vi "Configure Scaling.vi"(0 "Plugin_UI in":refnum<class "Plugin_UI.lvclass">, 11 "error in (no error)":errorcluster, 12 "Selected Channel":string) -> (4 "Plugin_UI out":refnum<class "Plugin_UI.lvclass">, 6 "Scale Active?":bool, 15 "error out":errorcluster)   [LabVIEW 2020, in "Plugin.lvlib" / "Plugin_UI.lvclass"]
doc: "Extracts all the measurement channels and display it in the Scale Settings window. Once the Scale settings window is closed, the scalling information of all the active channel is replaced with latest information from Scale Settings VI."
uses:
  Plugin_UI.lvclass
  C:/SVN_LabSys/labsys_lvcode/LabSys_SourceCode/builds/Libraries/LabSys Framework.lvlibp/Configurable Data Node/Configuration Interface/Configuration Interface.lvclass
  Plugin_UI.lvclass/Plugin_UI.ctl
  Read Input Channels[].vi
  Write Input Channels[].vi
  builds/Libraries/LabSys Framework.lvlibp/Configurable Data Node/Configuration Interface/Read Module Configuration.vi
  Read Scaling Functions.vi
  Read Lookup Tables.vi
  Write Scaling Functions.vi
  Write Lookup Tables.vi
  Channels/Input Channels/Input Channels.lvclass
  builds/Libraries/LabSys Framework.lvlibp/Configuration Storage/Module Configuration/Module Configuration.lvclass
  builds/Libraries/Shared GUI Library.lvlibp/Shared GUI Library/Scale Settings Dialog/Scale Settings Dialog.lvlib
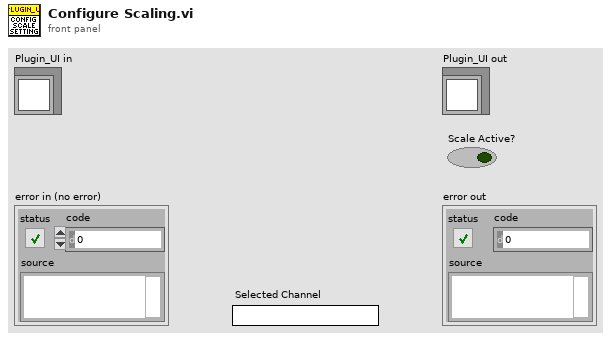
[diagram p1: front panel]
types:
  T1 = typedef "LabSys Framework.lvlibp/Configuration Storage.lvlib/Test Configuration.lvclass/Function Information.ctl" = cluster{"Name":string, "Expression":string, "Constants":T2[], "Test Data":dbl[][]}
  T2 = typedef "LabSys Framework.lvlibp/Configuration Storage.lvlib/Test Configuration.lvclass/Function Constant Value.ctl" = cluster{"Constant Name":string, "Value":dbl}
  T3 = typedef "LabSys Framework.lvlibp/Configuration Storage.lvlib/Test Configuration.lvclass/Table Information.ctl" = cluster{"Name":string, "Lookup Table":dbl[][]}
  T4 = typedef "LabSys Framework.lvlibp/Configuration Storage.lvlib/Test Configuration.lvclass/Channel Information.ctl" = cluster{"Channel Direction":T5, "Alias":string, "Refresh (ms)":dbl, "Scaling Information":T6, "Value Type":T8, "Subchannels":T9[], "Auxiliary Data":variant, "Group":i32}
  T5 = typedef "LabSys Framework.lvlibp/Configuration Storage.lvlib/Test Configuration.lvclass/Channel Directions.ctl" = enum8{"Module Input", "Module Output"}
  T6 = typedef "LabSys Framework.lvlibp/Configuration Storage.lvlib/Test Configuration.lvclass/Scaling Information.ctl" = cluster{"Active":bool, "Scaling Type":T7, "Output Minimum":dbl, "Output Maximum":dbl, "Raw Minimum":dbl, "Raw Maximum":dbl, "Output Unit":string, "Function":string, "Lookup Table":string}
  T7 = typedef "LabSys Framework.lvlibp/Configuration Storage.lvlib/Test Configuration.lvclass/Scaling Types.ctl" = enum8{"Linear", "Function", "Lookup Table"}
  T8 = typedef "Framework Base Library.lvlibp/Value Types.ctl" = enum8{"Unknown", "double", "double array", "Waveform", "DigWaveform", "Boolean", "Decimal", "String", "Db2Message", "Byte Array", "Unsigned Decimal"}
  T9 = typedef "LabSys Framework.lvlibp/Configuration Storage.lvlib/Test Configuration.lvclass/Subchannel Information.ctl" = cluster{"Alias":string, "Start Bit":u32, "Bit Length":u32, "Value Type":T8, "Auxiliary Data":variant}
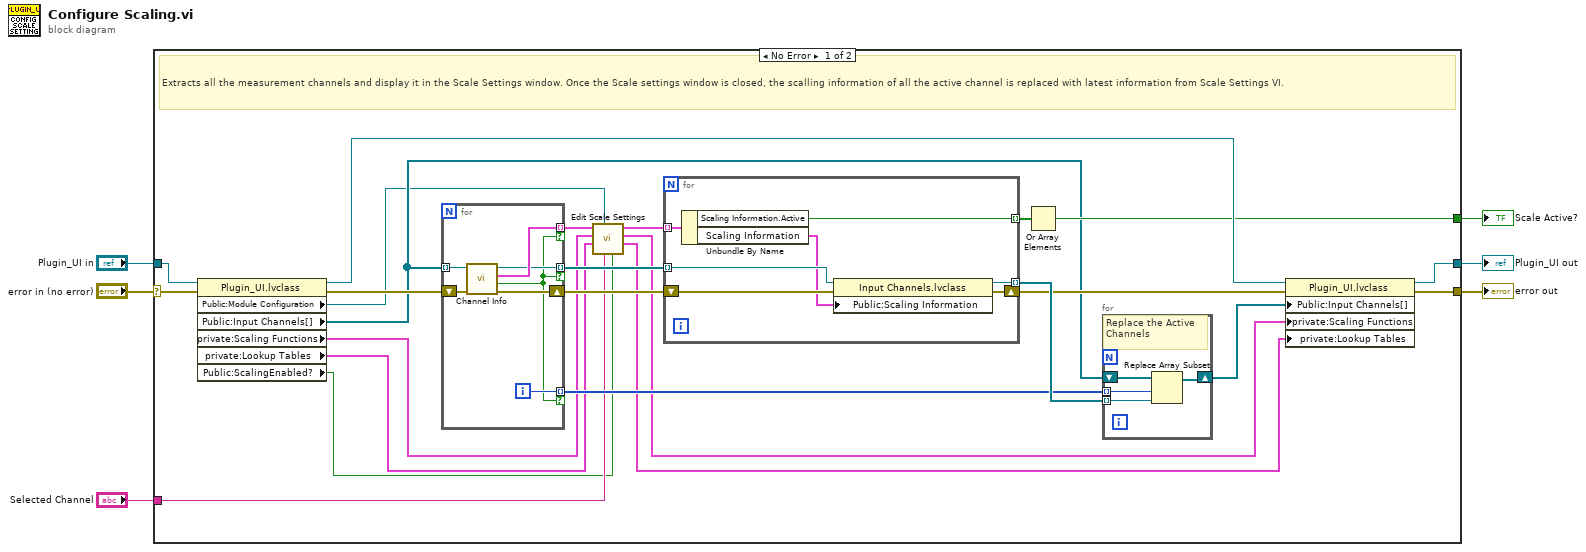
[diagram p0: block diagram]
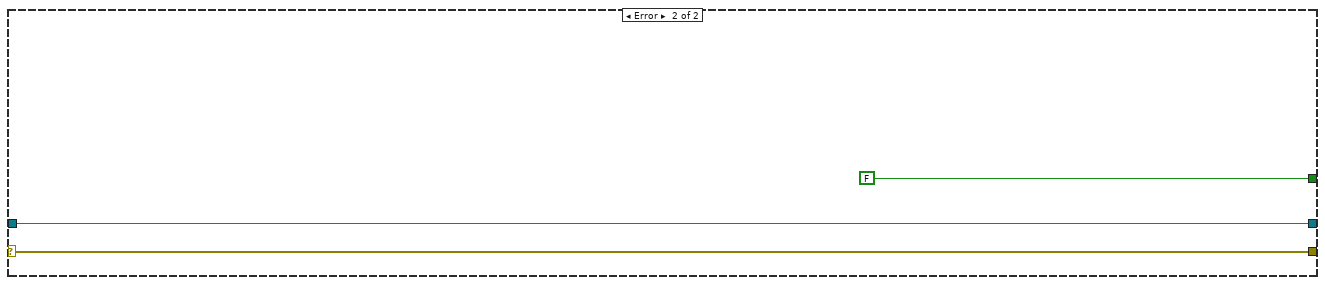
[diagram p2: hidden frame]
diagram:
  n1 = case shown="No Error" "error in (no error)" {
    selector: "error in (no error)" -> [w15 w51]
    tunnel: [w20 FALSE] -> w6
    tunnel: [w18 w50] -> w5
    tunnel: "Plugin_UI in" -> [w17 w50]
    tunnel: [w16 w51] -> w3
    tunnel: "Selected Channel" -> [w10 _]
    frame No Error {
      # "Extracts all the measurement channels and display it in the Scale Settings window. Once the Scale settings window is closed, the scalling information of all the active channel is replaced with latest information from Scale Settings VI."
      n2 = property class="Plugin_UI.lvclass"(reference=w17, error in=w15) -> (reference out=w27:refnum<class "Plugin_UI.lvclass">, error out=w22:errorcluster, "Public:Module Configuration"=w11:refnum<class "Module Configuration.lvclass">, "Public:Input Channels[]"=w12:refnum<class "Input Channels.lvclass">[], "private:Scaling Functions"=w14:T1[], "private:Lookup Tables"=w13:T3[], "Public:ScalingEnabled?"=w7:bool)
      n3 = for {
        shift-right: [w40] -> w24
        shift-left: w22 -> [w41]
        tunnel: w12 -> [w39] mode=indexing
        tunnel: [w38] -> w23 mode=indexing if=w35
        tunnel: [w37] -> w26 mode=indexing if=w35
        tunnel: [w36] -> w29 mode=indexing if=w35
        i -> [w36]
        n4 = call-dynamic "Channel Info.vi"("error in"=w41, "Input Channels in"=w39) -> ("error out"=w40:errorcluster, "Channel Active?"=w35:bool, "Channel Information"=w38:T4, "Input Channels out"=w37:refnum<class "Input Channels.lvclass">)  [unwired: 6 in]
      }
      n5 = call "Edit Scale Settings.vi"("Enable Editing"=w7, "Selected Channel"=w10, "Module Configuration"=w11, "Lookup Tables in"=w13, "Scaling Functions in"=w14, "Channel Information in"=w23) -> ("Lookup Tables out"=w8:T3[], "Scaling Functions out"=w9:T1[], "Channel Information out"=w21:T4[])  [unwired: 3 in]
      n6 = for {
        tunnel: w21 -> [w48] mode=indexing
        tunnel: [w47] -> w19 mode=indexing
        shift-right: [w45] -> w25
        shift-left: w24 -> [w46]
        tunnel: w26 -> [w44] mode=indexing
        tunnel: [w42] -> w30 mode=indexing
        n7 = Unbundle By Name(w48) -> ("Scaling Information.Active"=w47:bool, "Scaling Information"=w43:T6)
        n8 = property class="Input Channels.lvclass"(reference=w44, error in=w46, "Public:Scaling Information"=w43) -> (reference out=w42:refnum<class "Input Channels.lvclass">, error out=w45:errorcluster)
      }
      n9 = Or Array Elements(Boolean array=w19) -> (logical OR=w20:bool)
      n10 = for {
        tunnel: w30 -> [w34] mode=indexing
        tunnel: w29 -> [w33] mode=indexing
        shift-right: [w31] -> w28
        shift-left: w12 -> [w32]
        # "Replace the Active Channels"
        n11 = Replace Array Subset(array=w32, new element=w34, index=w33) -> (w31:refnum<class "Input Channels.lvclass">[])
      }
      n12 = property class="Plugin_UI.lvclass"(reference=w27, error in=w25, "Public:Input Channels[]"=w28, "private:Scaling Functions"=w9, "private:Lookup Tables"=w8) -> (reference out=w18:refnum<class "Plugin_UI.lvclass">, error out=w16:errorcluster)
    }
    frame Error {
    }
  }
  "Scale Active?" <- w6
  "Plugin_UI out" <- w5
  "error out" <- w3
